vi "BDDOP300.vi"(8 "errin":errorcluster, 10 "DATA IN":T1) -> (0 "error out":errorcluster, 3 "chaîne concaténée":string)   [LabVIEW 2020]
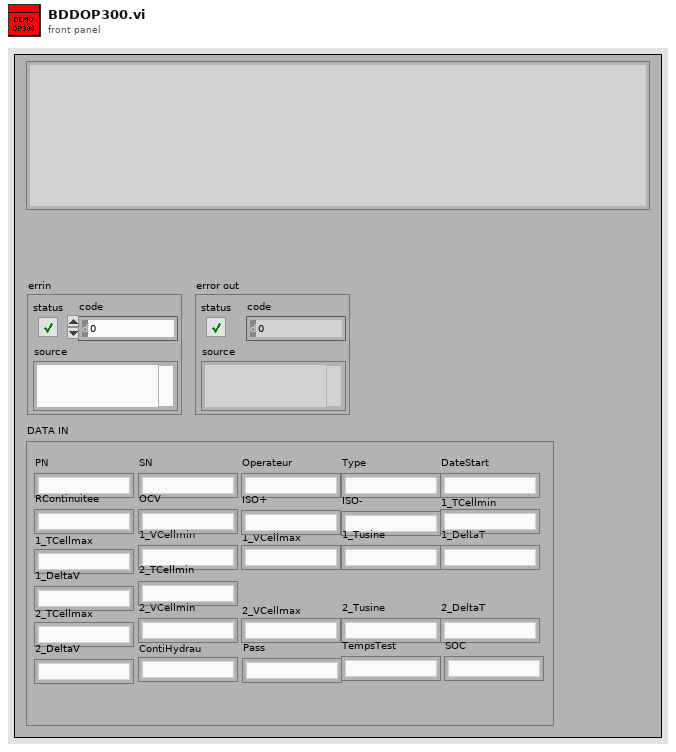
[diagram p1: front panel]
types:
  T1 = cluster{"PN":string, "SN":string, "Operateur":string, "Type":string, "DateStart":string, "RContinuitee":string, "OCV":string, "ISO+":string, "ISO-":string, "1_TCellmin":string, "1_TCellmax":string, "1_VCellmin":string, "1_VCellmax":string, "1_Tusine":string, "1_DeltaT":string, "1_DeltaV":string, "2_TCellmin":string, "2_TCellmax":string, "2_VCellmin":string, "2_VCellmax":string, "2_Tusine":string, "2_DeltaT":string, "2_DeltaV":string, "ContiHydrau":string, "Pass":string, "TempsTest":string, "SOC":string}
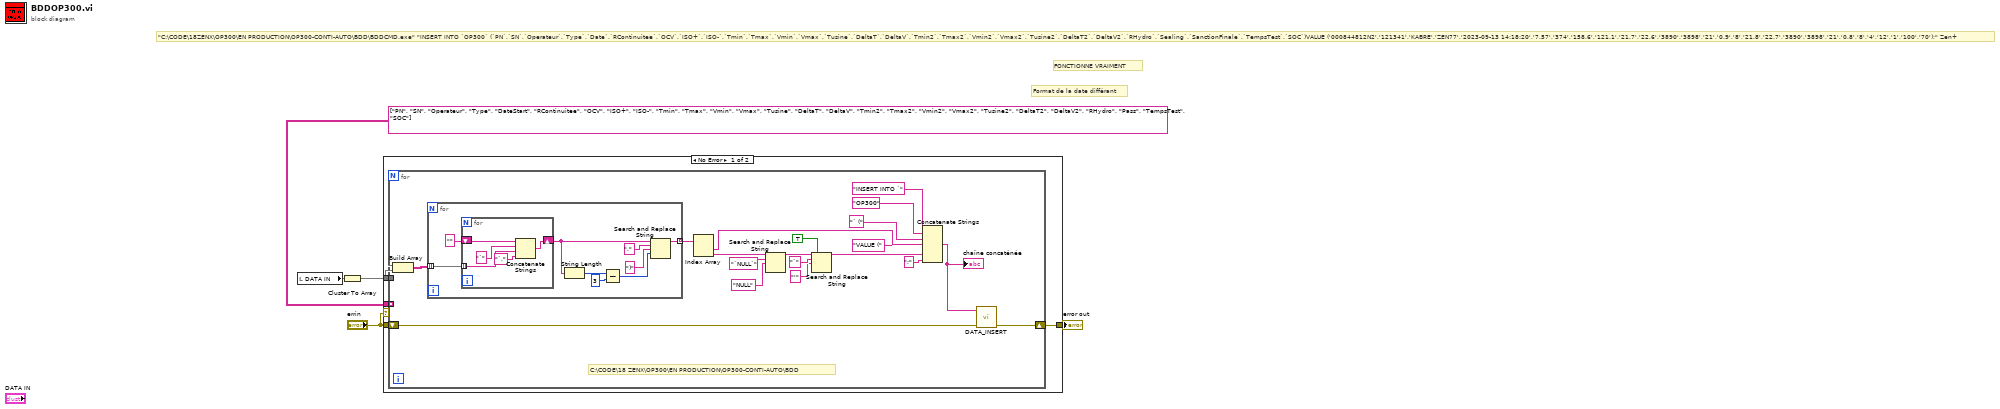
[diagram p0: block diagram]
diagram:
  # "FONCTIONNE VRAIMENT"
  # "\"C:\\CODE\\18ZENX\\OP300\\EN PRODUCTION\\OP300-CONTI-AUTO\\BDD\\BDDCMD.exe\" \"INSERT INTO `OP300` (`PN`,`SN`,`Operateur`,`Type`,`Date`,`RContinuitee`,`OCV`,`ISO+`,`ISO-`,`Tmin`,`Tmax`,`Vmin`,`Vmax`,`Tusine`,`DeltaT`,`DeltaV`,`Tmin2`,`Tmax2`,`Vmin2`,`Vmax2`,`Tusine2`,`DeltaT2`,`DeltaV2`,`RHydro`,`Sealing`,`SanctionFinale`,`TempsTest`,`SOC`)VALUE ('000844812N2','121341','KABRE','ZEN77','2023-09-13 14:18:20','7.57','374','158.6','121.1','21.7','22.6','3890','3898','21','0.9','8','21.8','22.7','3890','3898','21','0.8','8','4','12','1','100','70');\" Zen+"
  # "Format de la date différant"
  n1 = local read "DATA IN"() -> (w1:T1)
  n2 = Cluster To Array(cluster=w1) -> (array=w2:string[])
  n3 = case shown="No Error" "errin" {
    tunnel: "errin" -> [w9 w45]
    tunnel: [w8 w45] -> w5
    tunnel: string[][] [["PN", "SN", "Operateur", "Type", "DateStart", "RContinuitee", "OCV", "ISO+", "ISO-", "Tmin", "Tmax", "Vmin", "Vmax", "Tusine", "DeltaT", "DeltaV", "Tmin2", "Tmax2", "Vmin2", "Vmax2", "Tusine2", "DeltaT2", "DeltaV2", "RHydro", "Pass", "TempsTest", "SOC"]] -> [w7 _]
    tunnel: w2 -> [w6 _]
    frame No Error {
      n4 = for {
        shift-right: [w11] -> w8
        shift-left: w9 -> [w12]
        tunnel: w7 -> [w15] mode=indexing
        tunnel: w6 -> [w14]
        # "C:\\CODE\\18 ZENX\\OP300\\EN PRODUCTION\\OP300-CONTI-AUTO\\BDD"
        n5 = Build Array(w15, w14) -> (w30:string[][])
        n6 = for {
          tunnel: [w31] -> w16 mode=indexing
          tunnel: w30 -> [w39] mode=indexing
          n7 = for {
            shift-right: [w42] -> w32
            shift-left: "" -> [w41]
            tunnel: w39 -> [w40] mode=indexing
            n8 = Concatenate Strings(w41, "`" ("string"), w40, "`," ("string")) -> (w42:string)
          }
          n9 = String Length(string=w32) -> (length=w37:i32)
          n10 = Subtract(x=w37, y=3) -> (x-y=w35:i32)
          n11 = Search and Replace String(input string=w32, search string=",", replace string=")" ("replace string (\"\")"), offset=w35) -> (result string=w31:string)  [unwired: 4 in, 3 out]
        }
        n12 = Index Array(array=w16) -> (element #1=w26:string, element #2=w27:string)  [unwired: 2 in]
        n13 = Search and Replace String(input string=w27, search string="`NULL`", replace string="NULL" ("replace string (\"\")")) -> (result string=w28:string)  [unwired: 5 in, 3 out]
        n14 = Search and Replace String(replace all?=TRUE ("replace all? (F)"), input string=w28, search string="`", replace string="'" ("replace string (\"\")")) -> (result string=w29:string)  [unwired: 4 in, 3 out]
        n15 = Concatenate Strings("INSERT INTO `" ("string"), "OP300" ("chaîne"), "` (" ("string"), w26, "VALUE (" ("string"), w29, ";" ("string")) -> (w10:string)
        "chaîne concaténée" <- w10
        n16 = call <userlib>:"DATA_INSERT.vi"("errin"=w12, "INSERT"=w10) -> ("errout"=w11:errorcluster)  [unwired: 9 in]
      }
    }
    frame Error {
    }
  }
  "error out" <- w5
